vi "TestServer.vi"() -> ()   [LabVIEW 2021]
uses:
  AalborgServerModes.ctl
panel:
  in  "C:Dem(%)":dbl format="%#_13g"
  in  "Gas Release System":string="GRC-A"
  out "Output":cluster{"Start":dbl, "ServerMessages":string}[](array[cluster])
  in  "Multiplier":dbl=0.3
  in  "End":dbl=350.0
  in  "Start":dbl=1.0
  in  "Pause(s)":u32=5
  out "ServerMessages":string="\t\t\t\t\t\t\t\t\t\n"
  out "Q[Total]:Dem(l/min)":dbl min=0.0 max=360.0 step=1.0 format="%.2f"
  in  "Temperature channel":string="MFCcal:Temp:(C)"
  in  "Pressure channel":string="CSU:Pressure:mBar"
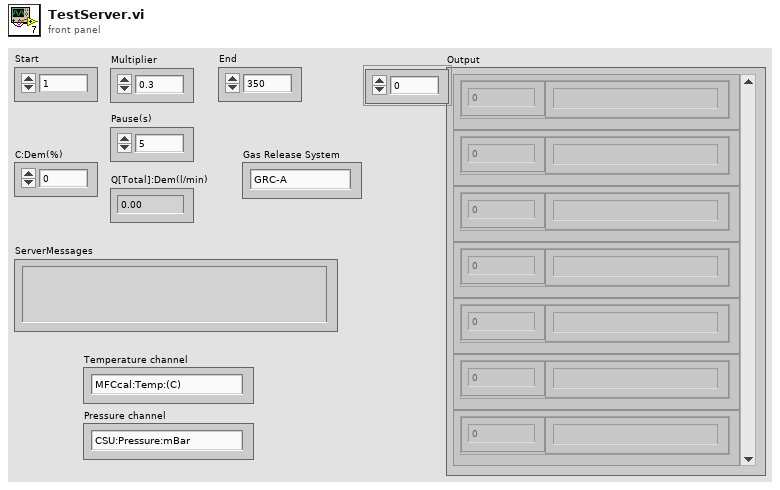
[diagram p1: front panel]
types:
  T1 = typedef "AalborgServerModes.ctl" = enum16{"Set Flows", "Check Flows Are Achievable", "Close All MFCs"}
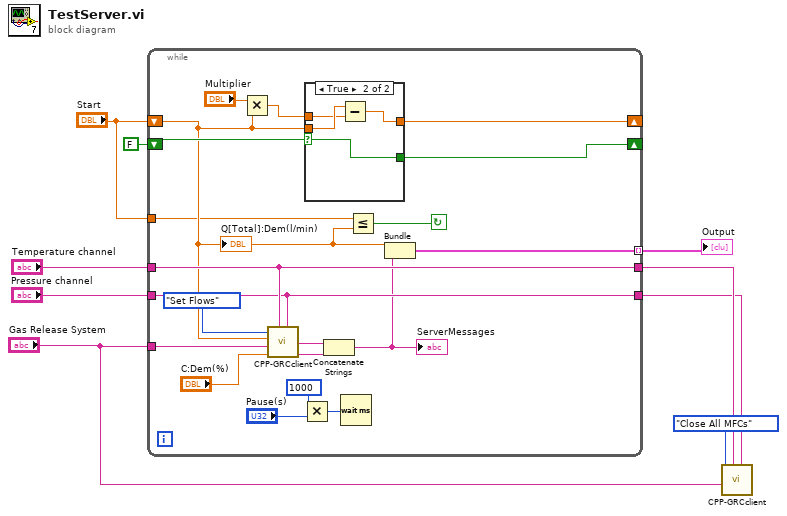
[diagram p0: block diagram]
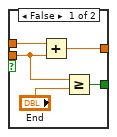
[diagram p2: hidden frame]
diagram:
  n1 = while {
    shift-right: [w27] -> _
    shift-left: "Start" -> [w14]
    tunnel: [w21] -> w9 mode=indexing
    tunnel: "Temperature channel" -> [w20]
    tunnel: [w20] -> w7
    tunnel: "Pressure channel" -> [w19]
    tunnel: [w19] -> w5
    tunnel: "Gas Release System" -> [w18]
    shift-right: [w16] -> _
    shift-left: FALSE -> [w17]
    tunnel: "Start" -> [w13]
    stop <- w15 continue-if-true
    n2 = Multiply(x="Multiplier", y=w14) -> (x*y=w28:dbl)
    n3 = call "CPP-GRCclient.vi"("Pressure channel"=w19, "Temperature channel"=w20, "C_dem:(%)"="C:Dem(%)", "Gas Release System"=w18, "Q_dem[Total]:(l/min)"=w14, "Mode"=AalborgServerModes."Set Flows") -> ("errorString"=w11:string, "infoString"=w12:string)  [unwired: 3 in, 1 out]
    n4 = Multiply(x=u32 1000, y="Pause(s)") -> (x*y=w23:u32)
    n5 = case shown="True" w17 {
      selector: w17 -> [_ w38]
      tunnel: w28 -> [w34 w35]
      tunnel: [w33 w37] -> w27
      tunnel: w14 -> [w31 w36]
      tunnel: [w30 w38] -> w16
      frame False {
        n6 = Add(x=w34, y=w31) -> (x+y=w33:dbl)
        n7 = Greater Or Equal?(x=w31, y="End") -> (x >= y?=w30:bool)
      }
      frame True {
        n8 = Subtract(x=w36, y=w35) -> (x-y=w37:dbl)
      }
    }
    n9 = Concatenate Strings(w12, w11) -> (w10:string)
    "ServerMessages" <- w10
    n10 = Wait (ms)(milliseconds to wait=w23) -> ()  [unwired: 1 out]
    n11 = Less Or Equal?(x=w13, y=w14) -> (x <= y?=w15:bool)
    n12 = Bundle("Start"=w14, w10) -> (w21:cluster{"Start":dbl, string})  [unwired: 1 in]
    "Q[Total]:Dem(l/min)" <- w14
  }
  "Output" <- w9
  n13 = call "CPP-GRCclient.vi"("Pressure channel"=w5, "Temperature channel"=w7, "Gas Release System"="Gas Release System", "Mode"=AalborgServerModes."Close All MFCs") -> ()  [unwired: 5 in, 3 out]
